vi "Save VI with XML Heaps With Overwrite Option.vi"(7 "Overwrite VI?":bool, 8 "error in (no error)":errorcluster, 10 "VI Path (temporary file)":path=path "", 11 "VI Refnum In":refnum<vi>) -> (0 "error out":errorcluster, 2 "VI Path out":path, 3 "VI Refnum Out":refnum<vi>)   [LabVIEW 2015]
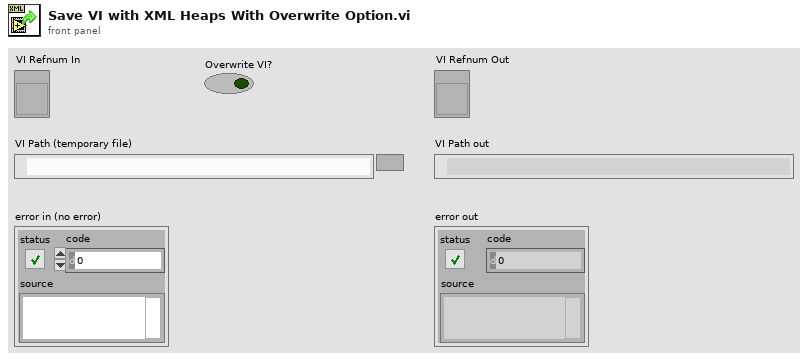
[diagram p1: front panel]
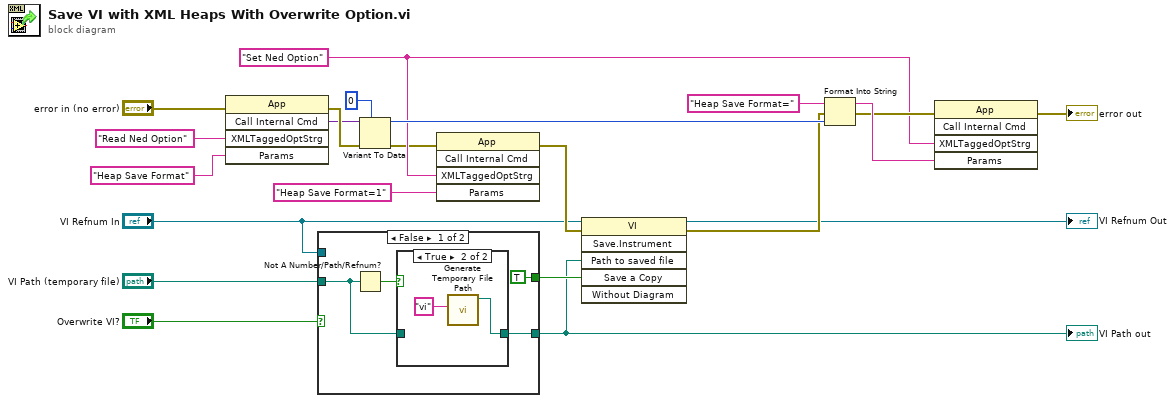
[diagram p0: block diagram]
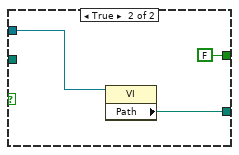
[diagram p3: hidden frame]
diagram:
  w13 = "Set Ned Option" ("Command Name")
  n1 = invoke class="App" method="Call Internal Cmd"(error in="error in (no error)", "XMLTaggedOptStrg"="Read Ned Option" ("Command Name"), "Params"="Heap Save Format") -> (error out=w22:errorcluster, "CallInternalCmd"=w19:variant)  [unwired: 2 in, 3 out]
  n2 = case shown="False" "Overwrite VI?" {
    tunnel: "VI Path (temporary file)" -> [w25 _]
    tunnel: [w24 w32] -> w1
    tunnel: "VI Refnum In" -> [_ w31]
    tunnel: [TRUE ("Save a Copy") FALSE ("Save a Copy")] -> w2
    frame False {
      n3 = Not A Number/Path/Refnum?(number/path/refnum=w25) -> (NaN/Path/Refnum?=w26:bool)
      n4 = case shown="True" w26 {
        tunnel: [w27 w29] -> w24
        tunnel: w25 -> [w27 _]
        frame False {
        }
        frame True {
          n5 = call <vilib>:"Generate Temporary File Path.vi"("Temporary File Extension (tmp)"="vi") -> ("Unique Temporary File Path"=w29:path)  [unwired: 9 in, 1 out]
        }
      }
    }
    frame True {
      n6 = property class="VI"(reference=w31) -> ("Path"=w32:path)  [unwired: 1 in, 2 out]
    }
  }
  "VI Path out" <- w1
  n7 = Variant To Data(error in=w22, type=0, Variant=w19) -> (data=w16:i32, error out=w12:errorcluster)
  n8 = invoke class="App" method="Call Internal Cmd"(error in=w12, "XMLTaggedOptStrg"=w13, "Params"="Heap Save Format=1") -> (error out=w10:errorcluster)  [unwired: 2 in, 4 out]
  n9 = invoke class="VI" method="Save.Instrument"(reference="VI Refnum In", error in=w10, "Path to saved file"=w1, "Save a Copy"=w2) -> (reference out=→"VI Refnum Out":refnum<vi>, error out=w9:errorcluster)  [unwired: 2 in, 4 out]
  n10 = Format Into String(initial string="Heap Save Format=", error in=w9, w16) -> (resulting string=w15:string, error out=w14:errorcluster)  [unwired: 1 in]
  n11 = invoke class="App" method="Call Internal Cmd"(error in=w14, "XMLTaggedOptStrg"=w13, "Params"=w15) -> (error out=→"error out":errorcluster)  [unwired: 2 in, 4 out]
